vi "LIDAR Present Variable.vi"() -> ()   [LabVIEW 2014]
panel:
  in  "LIDAR Present":bool
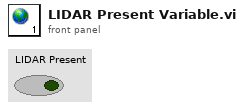
[diagram p1: front panel]
diagram:
